vi "Get_Device_ID.vi"(8 "错误输入":errorcluster) -> (0 "错误输出":errorcluster, 3 "Device_ID":string)   [LabVIEW 2020]
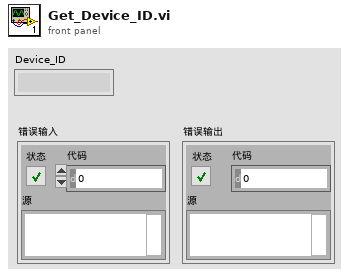
[diagram p1: front panel]
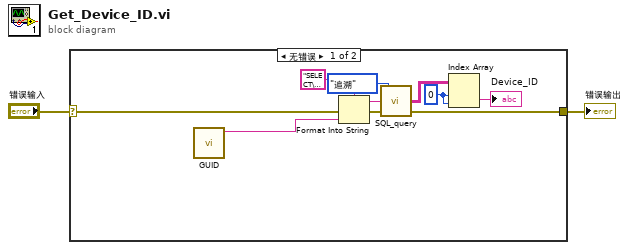
[diagram p0: block diagram]
diagram:
  n1 = case shown="无错误" "错误输入" {
    selector: "错误输入" -> [w9 w13]
    tunnel: [w7 w13] -> w1
    frame No Error {
      w11 = 0 ("索引 (行)")
      n2 = call "GUID.vi"() -> ("trimmed string"=w4:string)  [unwired: 11 in]
      n3 = Format Into String(format string="SELECT\ndbo.Device.DEVICE_ID\n\nFROM\ndbo.Device\nWHERE\ndbo.Device.DEVICE_PC_ID = '%s'\n", error in=w9, w4) -> (resulting string=w12:string, error out=w8:errorcluster)  [unwired: 1 in]
      n4 = call "SQL_query.vi"("error in (no error)"=w8, "SQL query"=w12, "联机模式"=enum16{"单机", "追溯"}."追溯") -> ("error out"=w7:errorcluster, "data"=w6:string[][])  [unwired: 1 out]
      n5 = Index Array(array=w6, index (row)=w11, index (col)=w11) -> (element=→"Device_ID":string)
    }
    frame Error {
    }
  }
  "错误输出" <- w1
